vi "Map Tags to Channels.vi"(7 "instance id":string, 8 "error in (no error)":errorcluster, 9 "String Array":string[][](array[string]), 10 "Lines":T1[](array[typedef]), 11 "engine configuration in":refnum<class "engine configuration.lvclass">) -> (0 "error out":errorcluster, 3 "engine configuration out":refnum<class "engine configuration.lvclass">)   [LabVIEW 2015, in "Increment editor node.lvclass"]
uses:
  Increment editor node.lvclass
  module/configuration/Line.ctl
  <vilib>/NI/Tag Bus Module Framework/channel/TBM channel.lvclass
  <vilib>/NI/Module Execution Interface/Engine Configuration/engine configuration.lvclass
  module/configuration/Increment configuration.lvclass
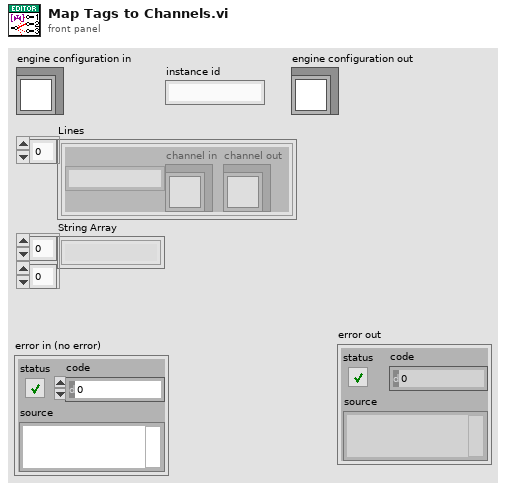
[diagram p1: front panel]
types:
  T1 = typedef "Increment configuration.lvclass/Line.ctl" = cluster{"Name":string, "channel in":refnum<class "TBM channel.lvclass">, "channel out":refnum<class "TBM channel.lvclass">}
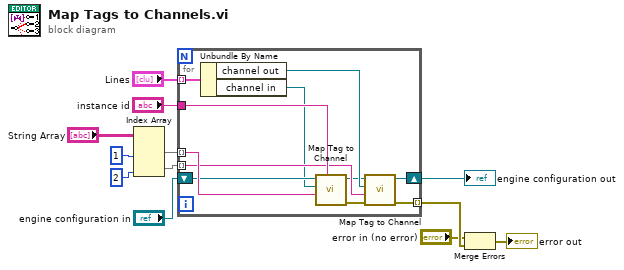
[diagram p0: block diagram]
diagram:
  n1 = Index Array(array="String Array", index (col) #1=1 ("disabled index (col)"), index (col) #2=2 ("index (col)")) -> (element #1=w6:string[], element #2=w1:string[])  [unwired: 2 in]
  n2 = for {
    tunnel: "Lines" -> [w23] mode=indexing
    tunnel: w6 -> [w21] mode=indexing
    shift-right: [w17] -> w9
    shift-left: "engine configuration in" -> [w16]
    tunnel: "instance id" -> [w22]
    tunnel: [w14] -> w11 mode=indexing
    tunnel: w1 -> [w20] mode=indexing
    n3 = Unbundle By Name(w23) -> ("channel out"=w19:refnum<class "TBM channel.lvclass">, "channel in"=w13:refnum<class "TBM channel.lvclass">)
    n4 = call "Map Tag to Channel.vi"("instance id"=w22, "Tag"=w21, "TBM channel in"=w13, "engine configuration in"=w16) -> ("error out"=w15:errorcluster, "engine configuration out"=w18:refnum<class "engine configuration.lvclass">)  [unwired: 6 in]
    n5 = call "Map Tag to Channel.vi"("error in (no error)"=w15, "Tag"=w20, "TBM channel in"=w19, "engine configuration in"=w18) -> ("error out"=w14:errorcluster, "engine configuration out"=w17:refnum<class "engine configuration.lvclass">)  [unwired: 6 in]
  }
  "engine configuration out" <- w9
  n6 = Merge Errors("error in (no error)", w11) -> (→"error out":errorcluster)
